vi "Read Item Path.vi"(8 "error in (no error)":errorcluster, 11 "ShortcutMenuSelectionMsg in":refnum<class "ShortcutMenuSelectionMsg.lvclass">) -> (0 "error out":errorcluster, 2 "Item Path":string, 3 "ShortcutMenuSelectionMsg out":refnum<class "ShortcutMenuSelectionMsg.lvclass">)   [LabVIEW 2020, in "MVA Framework.lvlib" / "ActorEvents.lvlib" / "ShortcutMenuSelectionMsg.lvclass"]
uses:
  ShortcutMenuSelectionMsg.lvclass
  ShortcutMenuSelectionMsg.lvclass/ShortcutMenuSelectionMsg.ctl
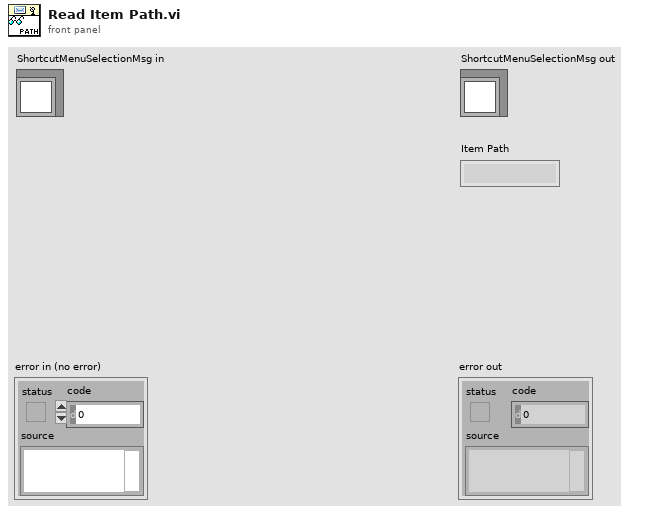
[diagram p1: front panel]
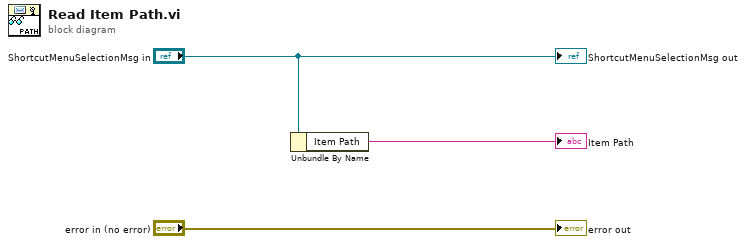
[diagram p0: block diagram]
diagram:
  n1 = Unbundle By Name("ShortcutMenuSelectionMsg in") -> ("Item Path"=→"Item Path":string)
  "error out" <- "error in (no error)"
  "ShortcutMenuSelectionMsg out" <- "ShortcutMenuSelectionMsg in"
